vi "Get Test Conditions.vi"(0 "Fuel":string(combo), 1 "CSV Array":string[][](array[string]), 3 "indices":T1, 5 "Oxidizer":string(combo), 9 "Diluent":string(combo), 11 "Equivalence Ratio":string(combo), 12 "Diluent Mole Fraction":string(combo), 13 "Initial Pressure":string(combo)) -> (4 "Test Found":bool, 6 "Fuel Partial Pressure":dbl, 8 "Test row":string[](array[string]), 10 "Oxidizer Partial Pressure":dbl, 15 "Diluent Partial Pressure":dbl)   [LabVIEW 2018]
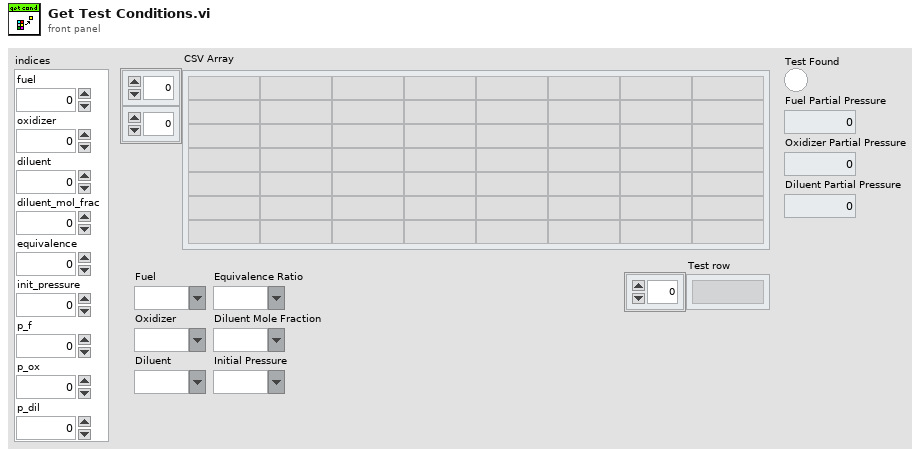
[diagram p1: front panel]
types:
  T1 = cluster{"fuel":i32, "oxidizer":i32, "diluent":i32, "diluent_mol_frac":i32, "equivalence":i32, "init_pressure":i32, "p_f":i32, "p_ox":i32, "p_dil":i32}
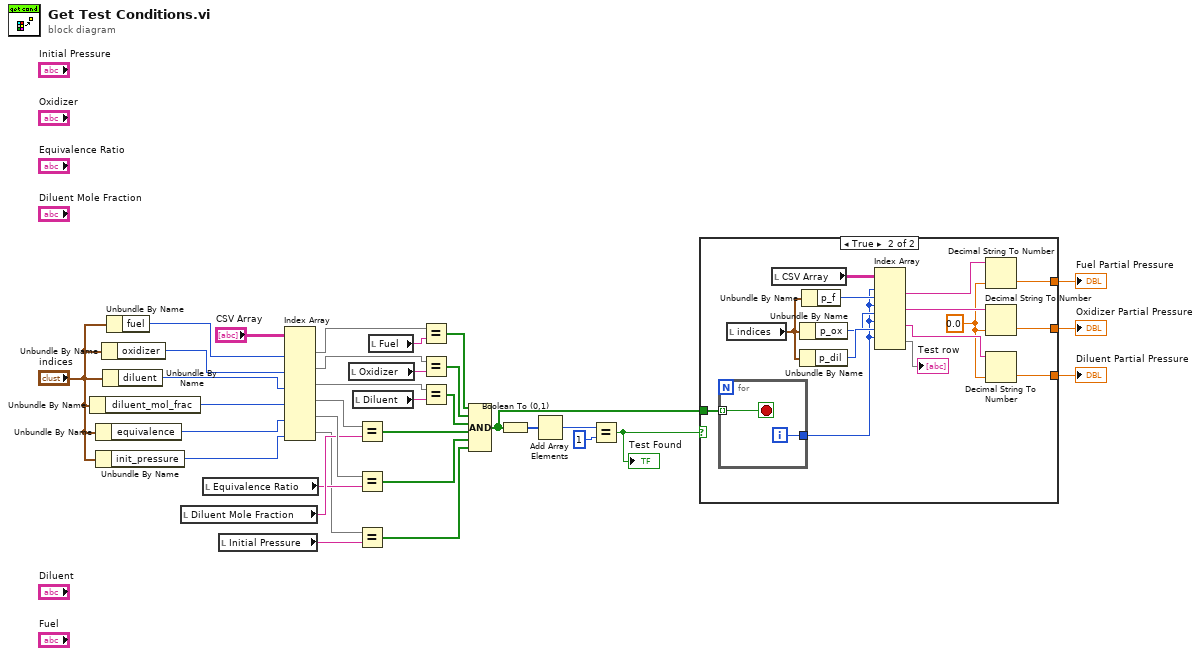
[diagram p0: block diagram]
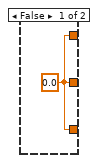
[diagram p2: hidden frame]
diagram:
  n1 = Unbundle By Name("indices") -> ("diluent_mol_frac"=w26:i32)
  n2 = Unbundle By Name("indices") -> ("equivalence"=w25:i32)
  n3 = Unbundle By Name("indices") -> ("init_pressure"=w9:i32)
  n4 = Unbundle By Name("indices") -> ("oxidizer"=w29:i32)
  n5 = Unbundle By Name("indices") -> ("diluent"=w27:i32)
  n6 = Unbundle By Name("indices") -> ("fuel"=w30:i32)
  n7 = local read "Diluent Mole Fraction"() -> (w16:string)
  n8 = local read "Equivalence Ratio"() -> (w15:string)
  n9 = local read "Initial Pressure"() -> (w7:string)
  n10 = Index Array(array="CSV Array", index (col) #1=w30, index (col) #2=w29, index (col) #3=w27, index (col) #4=w26, index (col) #5=w25, index (col) #6=w9) -> (element #1=w33:string[], element #2=w32:string[], element #3=w23:string[], element #4=w22:string[], element #5=w21:string[], element #6=w8:string[])  [unwired: 6 in]
  n11 = local read "Oxidizer"() -> (w31:string)
  n12 = local read "Diluent"() -> (w17:string)
  n13 = Equal?(x=w22, y=w16) -> (x = y?=w19:bool[])
  n14 = Equal?(x=w21, y=w15) -> (x = y?=w18:bool[])
  n15 = Equal?(x=w8, y=w7) -> (x = y?=w6:bool[])
  n16 = local read "Fuel"() -> (w34:string)
  n17 = Equal?(x=w33, y=w34) -> (x = y?=w28:bool[])
  n18 = Equal?(x=w32, y=w31) -> (x = y?=w24:bool[])
  n19 = Equal?(x=w23, y=w17) -> (x = y?=w20:bool[])
  n20 = Compound Arithmetic op=AND(w28, w24, w20, w19, w18, w6) -> (w10:bool[])
  n21 = Boolean To (0,1)(Boolean=w10) -> (0, 1=w14:i16[])
  n22 = Add Array Elements(numeric array=w14) -> (sum=w13:i16)
  n23 = Equal?(x=w13, y=i16 1) -> (x = y?=w11:bool)
  "Test Found" <- w11
  n24 = case shown="True" w11 {
    tunnel: w10 -> [_ w50]
    tunnel: [w35 w46] -> w5
    tunnel: [w35 w42] -> w4
    tunnel: [w35 w41] -> w3
    frame False {
      w35 = 0.0
    }
    frame True {
      w43 = 0.0
      n25 = for {
        tunnel: w50 -> [w52] mode=indexing
        tunnel: [w51] -> w37
        i -> [w51]
        stop <- w52 stop-if-true
      }
      n26 = local read "indices"() -> (w49:T1)
      n27 = local read "CSV Array"() -> (w48:string[][])
      n28 = Unbundle By Name(w49) -> ("p_ox"=w39:i32)
      n29 = Unbundle By Name(w49) -> ("p_dil"=w40:i32)
      n30 = Unbundle By Name(w49) -> ("p_f"=w38:i32)
      n31 = Index Array(array=w48, index (row) #1=w37, index (col) #1=w38, index (row) #2=w37, index (col) #2=w39, index (row) #3=w37, index (col) #3=w40, index (row) #4=w37) -> (element #1=w47:string, element #2=w44:string, element #3=w45:string, element #4=→"Test row":string[])  [unwired: 1 in]
      n32 = Decimal String To Number(string=w47, default (0L)=w43) -> (number=w46:dbl)  [unwired: 1 in, 1 out]
      n33 = Decimal String To Number(string=w44, default (0L)=w43) -> (number=w42:dbl)  [unwired: 1 in, 1 out]
      n34 = Decimal String To Number(string=w45, default (0L)=w43) -> (number=w41:dbl)  [unwired: 1 in, 1 out]
    }
  }
  "Diluent Partial Pressure" <- w3
  "Fuel Partial Pressure" <- w5
  "Oxidizer Partial Pressure" <- w4
